vi "GaugesFrontPanel.vi"() -> ()   [LabVIEW 2023]
uses:
  SlipIndicator.ctl
panel:
  in  "GPS/Baro_Vario":bool
  out "VarioNeedle":picture
  out "Compass Gauge":dbl(knob) scale=0.0..12.0 scale format="%#_1g"
  out "TurnBankPlanePicture":picture caption="Neue Grafik"
  in  "GPS/Mag":bool
  in  "GPS/Baro_Alt":bool
  out "TurnBankStdRate":bool
  in  "ScaleUnit(F=km/h; T=knots)":bool
  out "SpeedIndicatorNeedle":picture
  out "Heading Digital":dbl format="%.1f"
  out "Vario Digital":dbl format="%.1f"
  in  "ScaleUnit(F=m; T=feet)":bool
  out "AltNeedlePicture":picture
  out "Altitude digital":dbl
  out "GPS Data Valid?":bool
  out "GPS Sensor OK":bool
  out "UTC":string
  out "Local":string
  in  "Difference Local/UTC [h]":i32=1
  out "Inclinometer":T1 scale=-10.0..10.0
  out "ArtificialHorizon":picture
  # "AlfaJet"
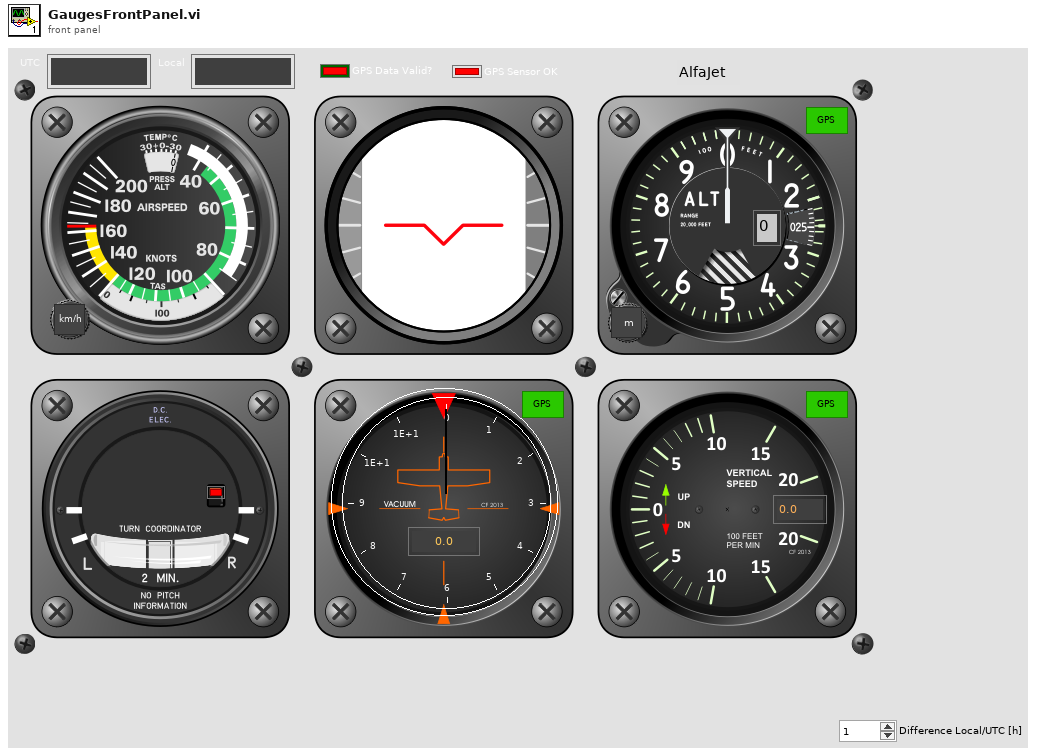
[diagram p1: front panel]
types:
  T1 = typedef "SlipIndicator.ctl" = dbl
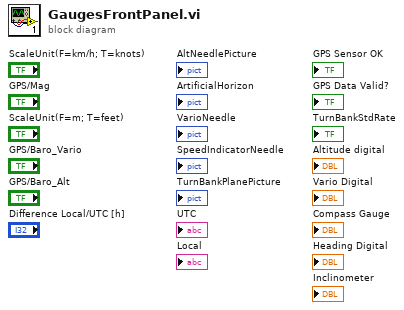
[diagram p0: block diagram]
diagram:
